vi "Software Update HCC Build EXE Locations.vi"(8 "Error In":errorcluster, 10 "Update Files (Option 1-24)":i32[](array[numeric]), 11 "Newfi Exe Folder Path":path) -> (0 "Error Out":errorcluster, 3 "Path Build List (Folder Locations)":path[](array[path]))   [LabVIEW 2016]
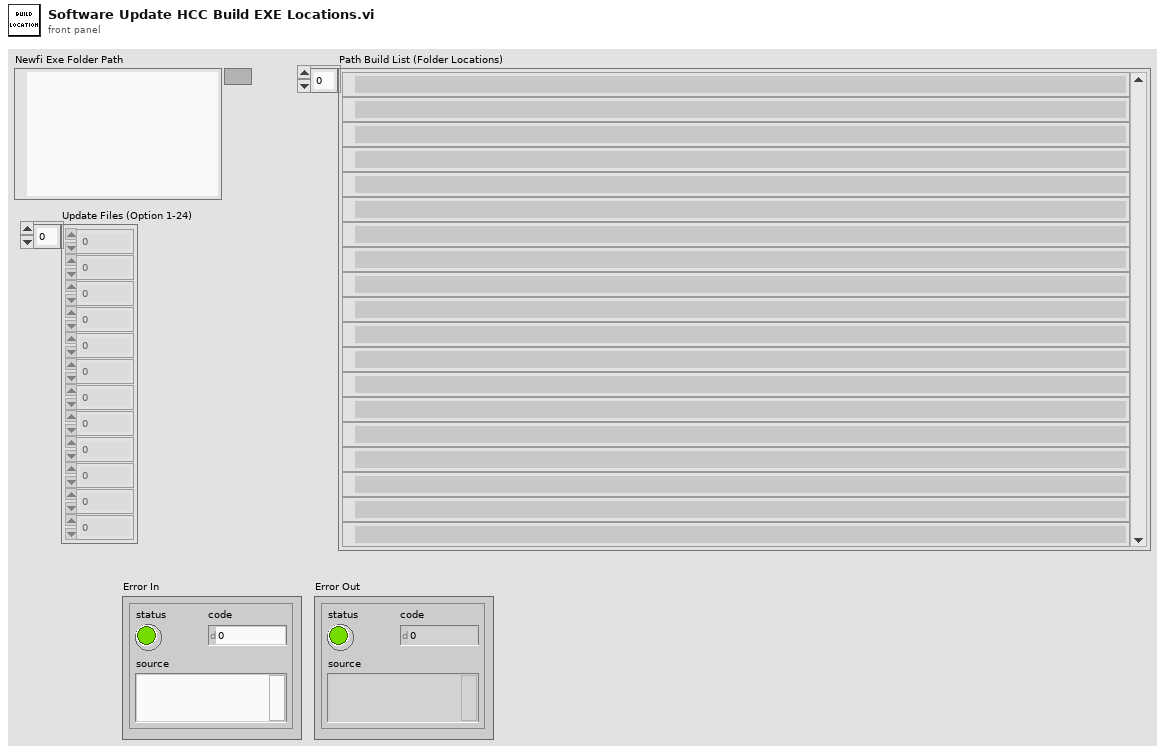
[diagram p1: front panel]
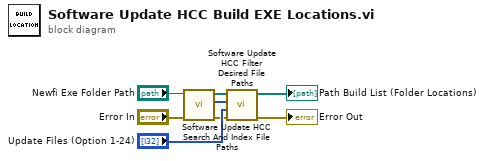
[diagram p0: block diagram]
diagram:
  n1 = call "Software Update HCC Search And Index File Paths.vi"("Error In"="Error In", "Newfi Exe Folder Path"="Newfi Exe Folder Path") -> ("Error Out"=w1:errorcluster, "Index of File Path"=w4:i32[], "File Path"=w5:path[])  [unwired: 7 in]
  n2 = call "Software Update HCC Filter Desired File Paths.vi"("Error In"=w1, "Update Files (Option 1-24)"="Update Files (Option 1-24)", "Index of File Path"=w4, "All File Paths"=w5) -> ("Error Out"=→"Error Out":errorcluster, "Desired File Paths"=→"Path Build List (Folder Locations)":path[])  [unwired: 6 in]
